vi "VI-Connect Reg Event Terminals To Pane.vi"(0 "VI in":refnum<vi>, 2 "Components":T1, 9 "Ref array":refnum<vi>, 11 "error in (no error)":errorcluster) -> (4 "VI out":refnum<vi>, 15 "error out":errorcluster)   [LabVIEW 2015]
uses:
  VI-Reg Event Components.ctl
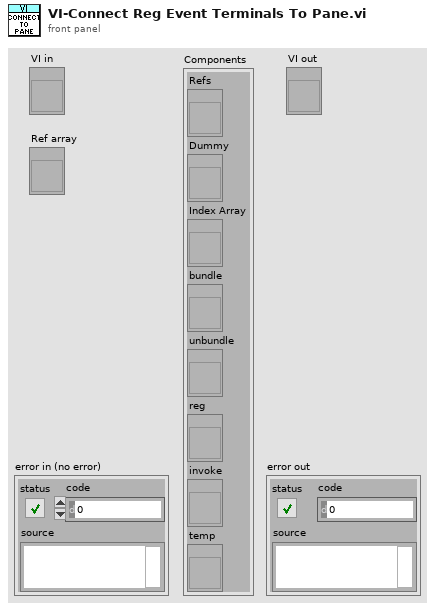
[diagram p1: front panel]
types:
  T1 = typedef "VI-Reg Event Components.ctl" = cluster{"Refs":refnum<vi>, "Dummy":refnum<vi>, "Index Array":refnum<vi>, "bundle":refnum<vi>, "unbundle":refnum<vi>, "reg":refnum<vi>, "invoke":refnum<vi>, "temp":refnum<vi>}
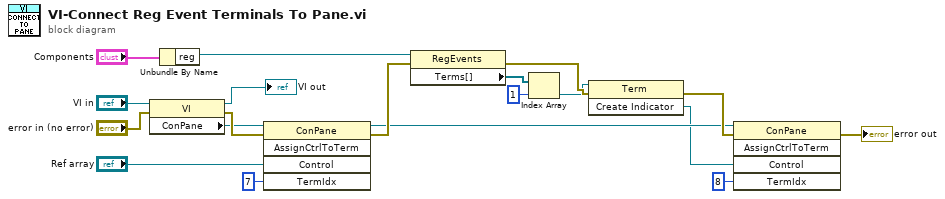
[diagram p0: block diagram]
diagram:
  n1 = property class="VI"(reference="VI in", error in="error in (no error)") -> (reference out=→"VI out":refnum<vi>, error out=w10:errorcluster, "ConPane"=w9:refnum<vi>)
  n2 = Unbundle By Name("Components") -> ("reg"=w14:refnum<vi>)
  n3 = invoke class="ConPane" method="AssignCtrlToTerm"(reference=w9, error in=w10, "Control"="Ref array", "TermIdx"=u32 7 ("Terminal Index")) -> (reference out=w4:refnum<vi>, error out=w18:errorcluster)  [unwired: 1 in, 3 out]
  n4 = property class="RegEvents"(reference=w14, error in=w18) -> (error out=w19:errorcluster, "Terms[]"=w15:refnum<vi>[])  [unwired: 1 out]
  n5 = Index Array(array=w15, index=1) -> (element=w17:refnum<vi>)
  n6 = invoke class="Term" method="Create Indicator"(reference=w17, error in=w19) -> (error out=w5:errorcluster, "Create Indicator"=w3:refnum<vi>)  [unwired: 1 in, 1 out]
  n7 = invoke class="ConPane" method="AssignCtrlToTerm"(reference=w4, error in=w5, "Control"=w3, "TermIdx"=u32 8 ("Terminal Index")) -> (error out=→"error out":errorcluster)  [unwired: 1 in, 4 out]
